vi "I2S PBDAT Out(David Documentation).vi"(0 "I2S.PBLRC IN":bool, 5 "I2S.Data":T1, 7 "Data Index":u16, 9 "Bit Count":u16, 11 "Word Length":u16) -> (4 "I2S.PBDAT OUT":bool)   [LabVIEW 2015]
uses:
  Audio Signals.ctl
panel:
  # "Overview: Write each bit of audio data to PBDAT pin."
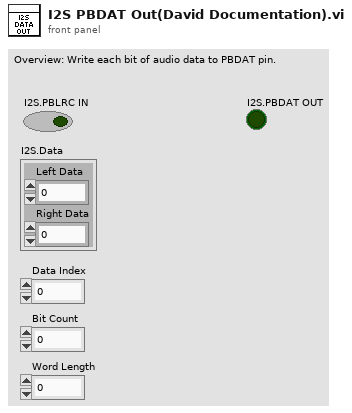
[diagram p1: front panel]
types:
  T1 = typedef "Audio Signals.ctl" = cluster{"Left Data":u32, "Right Data":u32}
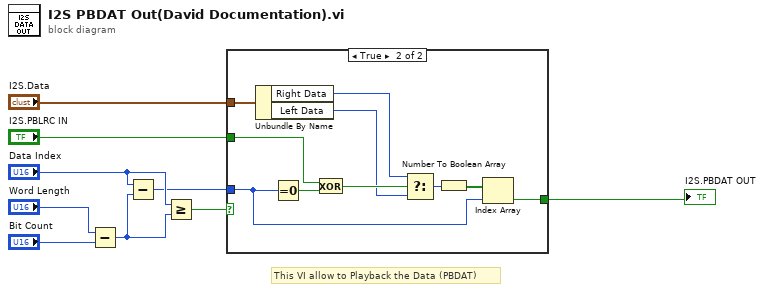
[diagram p0: block diagram]
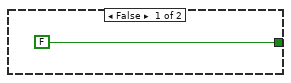
[diagram p2: hidden frame]
diagram:
  # "This VI allow to Playback the Data (PBDAT)"
  n1 = Subtract(x="Word Length", y="Bit Count") -> (x-y=w1:u16)
  n2 = Subtract(x="Data Index", y=w1) -> (x-y=w6:u16)
  n3 = Greater Or Equal?(x="Data Index", y=w1) -> (x >= y?=w8:bool)
  n4 = case shown="True" w8 {
    tunnel: [FALSE w14] -> w9
    tunnel: w6 -> [_ w13]
    tunnel: "I2S.Data" -> [_ w12]
    tunnel: "I2S.PBLRC IN" -> [_ w11]
    frame False {
    }
    frame True {
      n5 = Unbundle By Name(w12) -> ("Right Data"=w17:u32, "Left Data"=w16:u32)
      n6 = Equal To 0?(x=w13) -> (x = 0?=w19:bool)
      n7 = Exclusive Or(1:w19, 2:w11) -> (0:w18:bool)
      n8 = Select(t=w17, s=w18, f=w16) -> (s? t:f=w15:u32)
      n9 = Number To Boolean Array(number=w15) -> (Boolean array=w20:bool[])
      n10 = Index Array(array=w20, index=w13) -> (element=w14:bool)
    }
  }
  "I2S.PBDAT OUT" <- w9
